vi "Post-Build Action.vi"(5 "Files Generated by Build":path[](array[path]), 6 "Top Level/Always Included VIs":path[](array[path]), 7 "Destination Path":path, 8 "error in (no error)":errorcluster, 9 "Target Name":string, 10 "Build Specification Name":string, 11 "Project Path":path) -> (0 "error out":errorcluster)   [LabVIEW 2024]
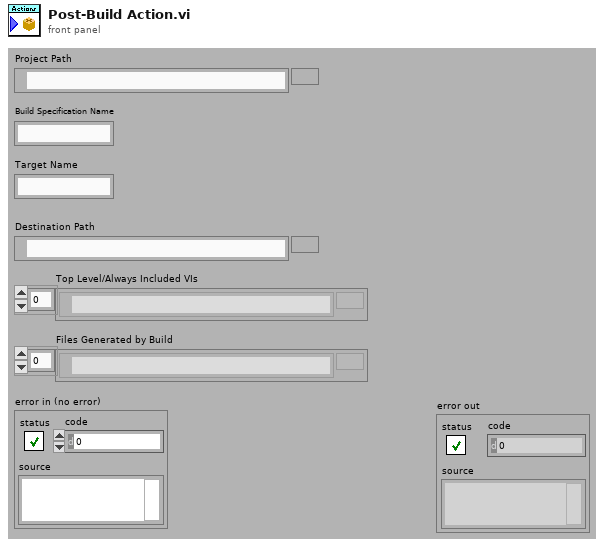
[diagram p1: front panel]
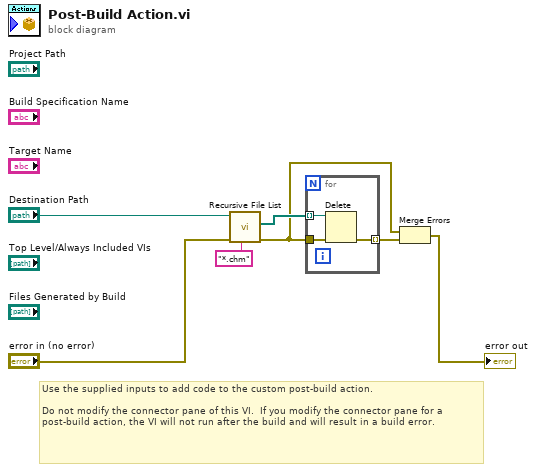
[diagram p0: block diagram]
diagram:
  # "Use the supplied inputs to add code to the custom post-build action.\n\nDo not modify the connector pane of this VI.  If you modify the connector pane for a post-build action, the VI will not run after the build and will result in a build error."
  n1 = call <vilib>:"Recursive File List.vi"("pattern"="*.chm", "error in (no error)"="error in (no error)", "Folder Path"="Destination Path") -> ("error out"=w1:errorcluster, "All Files in Dir"=w2:path[])  [unwired: 4 in, 3 out]
  n2 = for {
    tunnel: w2 -> [w10] mode=indexing
    tunnel: w1 -> [w9]
    tunnel: [w8] -> w4 mode=indexing
    n3 = Delete(path (use dialog)=w10, error in=w9) -> (error out=w8:errorcluster)  [unwired: 3 in, 2 out]
  }
  n4 = Merge Errors(w1, w4) -> (→"error out":errorcluster)
